vi "PPR_DRIVE_EXECUTE.vi"(6 "Pass_Through_Time":dbl=-1.0 format="%33.4f", 8 "error in (no error)":errorcluster) -> (0 "error out":errorcluster)   [LabVIEW 2019]
uses:
  <vilib>/Rock Robotics/WPI/ThirdParty/JAS_Junk/TrajLib/VI/BoolCmd_Recv_Internal.vi
  <vilib>/Rock Robotics/WPI/ThirdParty/JAS_Junk/TrajLib/VI/numCmd_ObtainQueue_TwoDbl.vi
  <vilib>/Rock Robotics/WPI/ThirdParty/JAS_Junk/TrajLib/VI/Util_GetTime_U32.vi
  <vilib>/Rock Robotics/WPI/ThirdParty/JAS_Junk/TrajLib/MathUtil_InputModulus.vi
  <vilib>/Rock Robotics/WPI/ThirdParty/JAS_Junk/TrajLib/VI/BoolCmd_ObtainQueue.vi
  <vilib>/Rock Robotics/WPI/ThirdParty/JAS_Junk/TrajLib/VI/Util_GetTime_U64.vi
  PPR_DRIVE_GLOBALS.vi
  <vilib>/Rock Robotics/WPI/ThirdParty/JAS_Junk/TrajLib/Trajectory_Library.lvlib
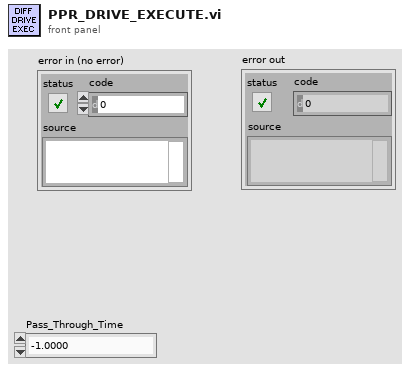
[diagram p1: front panel]
types:
  T1 = typedef "WPI_GyroDevRef.ctl" = cluster{"DevStatus":errorcluster, "Analog Channel":T2, "Gain (VoltsPerDegree/Second)":dbl, "Gyro Type":enum16{"Analog", "XRS450"}, "Handle":i32, "SPI Bus":T3, "Device Found":bool, "Sample Rate":dbl, "Calibrate On Open":bool, "Offset":dbl}
  T2 = typedef "FPGA_AIChannel.ctl" = enum8{"AI 0", "AI 1", "AI 2", "AI 3", "AI MXP 0", "AI MXP 1", "AI MXP 2", "AI MXP 3", "Invalid"}
  T3 = typedef "spi_bus.ctl" = enum16{"SPI On-Board, CS0", "SPI On-Board, CS1", "SPI On-Board, CS2", "SPI On-Board, CS3", "SPI MXP", "Invalid"}
  T4 = typedef "PPR_DRIVE_Wheel_TYPDEF.ctl" = cluster{"Drive Motor":T5, "Wheel Encoder":T10}
  T5 = typedef "WPI_MotorControlDeviceRef.ctl" = cluster{"DeviceStatus":errorcluster, "Type":T6, "PWM":cluster{"PWM Channel":T7, "DeadBand":T8}, "CAN":cluster{"Device Number":u8, "SetOutput VI Ref":variant, "GetOutput VI Ref":variant, "Enable VI Ref":variant, "Disable VI Ref":variant, "Data":variant}, "Invert":bool, "DIO PWM":cluster{"PWM \"Enable\" Channel":T7, "DIOChannel":T9, "PWM Rate":dbl}}
  T6 = typedef "WPI_MotorControlType.ctl" = enum16{"PWM", "CAN", "DIO PWM"}
  T7 = typedef "FPGA_DIOPWMChannel.ctl" = enum8{"PWM 0", "PWM 1", "PWM 2", "PWM 3", "PWM 4", "PWM 5", "PWM 6", "PWM 7", "PWM 8", "PWM 9", "PWM MXP 0", "PWM MXP 1", "PWM MXP 2", "PWM MXP 3", "PWM MXP 4", "PWM MXP 5", "PWM MXP 6", "PWM MXP 7", "PWM MXP 8", "PWM MXP 9", "Invalid"}
  T8 = typedef "WPI_PWMDeadband.ctl" = cluster{"Name":string, "maxPositivePwm":i32, "minPositivePwm":i32, "centerPwm":i32, "maxNegativePwm":i32, "minNegativePwm":i32, "angularRange":u16}
  T9 = typedef "FPGA_DIOChannel.ctl" = enum8{"DIO 0", "DIO 1", "DIO 2", "DIO 3", "DIO 4", "DIO 5", "DIO 6", "DIO 7", "DIO 8", "DIO 9", "DIO MXP 0", "DIO MXP 1", "DIO MXP 2", "DIO MXP 3", "DIO MXP 4", "DIO MXP 5", "DIO MXP 6", "DIO MXP 7", "DIO MXP 8", "DIO MXP 9", "DIO MXP 10", "DIO MXP 11", "DIO MXP 12", "DIO MXP 13", "DIO MXP 14", "DIO MXP 15", "SPI Port CS1", "SPI Port CS2", "SPI Port CS3", "SPI Port MISO", "SPI Port MOSI", "Invalid"}
  T10 = typedef "WPI_EncoderDevRef.ctl" = cluster{"DevStatus":errorcluster, "EncoderIndex":T11, "CounterIndex":T12, "DistancePerCount":dbl, "Decoding Type":T13}
  T11 = typedef "FPGA_EncoderIdx.ctl" = enum8{"Enc 0", "Enc 1", "Enc 2", "Enc 3", "Enc 4", "Enc 5", "Enc 6", "Enc 7", "Invalid"}
  T12 = typedef "FPGA_CounterCtrSystemIndex.ctl" = enum8{"Ctr 0", "Ctr 1", "Ctr 2", "Ctr 3", "Ctr 4", "Ctr 5", "Ctr 6", "Ctr 7", "Invalid"}
  T13 = typedef "WPI_EncoderType.ctl" = enum16{"1x", "2x", "4x"}
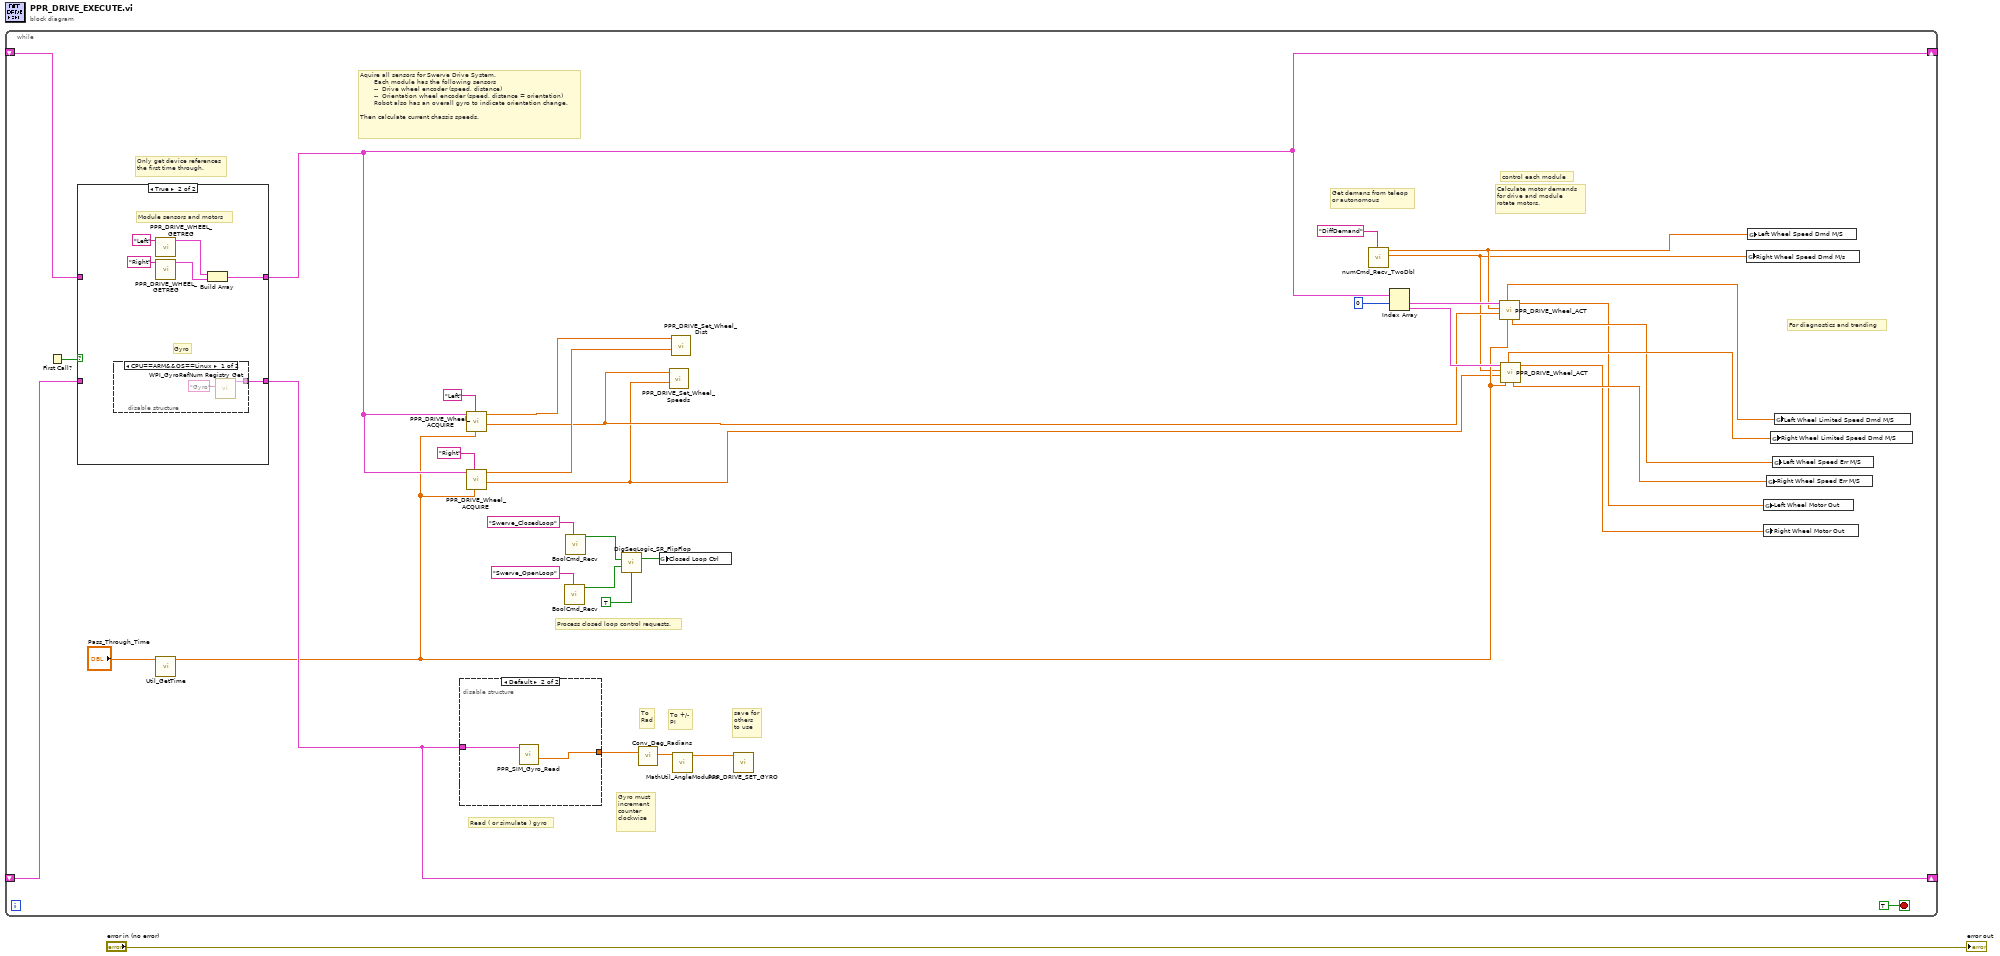
[diagram p0: block diagram]
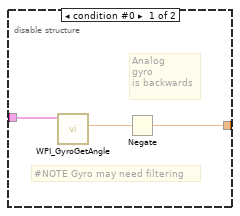
[diagram p4: hidden frame]
diagram:
  n1 = while {
    shift-right: [w25] -> _
    shift-left: _ -> [w26]
    shift-right: [w24] -> _
    shift-left: _ -> [w23]
    stop <- TRUE stop-if-true
    # "Process closed loop control requests."
    # "Only get device references\nthe first time through."
    # "save for\nothers\nto use"
    # "For diagnostics and trending"
    # "Gyro must\nincrement \ncounter\nclockwise"
    # "To +/-\nPI"
    # "To\nRad"
    # "Read ( or simulate ) gyro"
    # "Aquire all sensors for Swerve Drive System.\n       Each module has the following sensors\n       --  Drive wheel encoder (speed, distance)\n       --  Orientation wheel encoder (speed, distance = orientation)\n       Robot also has an overall gyro to indicate orientation change.\n\nThen calculate current chassis speeds."
    # "Calculate motor demands\nfor drive and module \nrotate motors."
    # "Get demans from teleop\nor autonomous"
    # "control each module"
    n2 = First Call?() -> (First Call?: T/F=w27:bool)
    n3 = case shown="True" w27 {
      tunnel: [w38 w42] -> w25
      tunnel: [w37 w41] -> w24
      tunnel: w26 -> [w38 _]
      tunnel: w23 -> [w37 _]
      frame False {
      }
      frame True {
        # "Module sensors and motors"
        # "Gyro"
        n4 = disable-structure shown="CPU==ARM&&OS==Linux" {
          disable-tunnel: [w45 _] -> w41
          frame condition #0 {
            n5 = call <vilib>:"WPI_GyroRefNum Registry Get.vi"("refnum name"="Gyro") -> ("GyroDevRef"=w45:T1)  [unwired: 9 in, 1 out]
          }
          frame condition #1 (active) {
          }
        }
        n6 = call "PPR_DRIVE_WHEEL_GETREG.vi"("Side"="Left") -> ("Diff Wheel TypDef"=w43:T4)  [unwired: 10 in]
        n7 = call "PPR_DRIVE_WHEEL_GETREG.vi"("Side"="Right") -> ("Diff Wheel TypDef"=w44:T4)  [unwired: 10 in]
        n8 = Build Array(w43, w44) -> (w42:T4[])
      }
    }
    n9 = call <vilib>:"Util_GetTime.vi"("Pass_Through_Time"="Pass_Through_Time") -> ("FPGA_Time_Seconds"=w22:dbl)  [unwired: 8 in, 2 out]
    n10 = disable-structure shown="Default" {
      disable-tunnel: w24 -> [w49 w51]
      disable-tunnel: [w47 w50] -> w30
      frame condition #0 {
        # "Analog\ngyro\nis backwards"
        # "#NOTE Gyro may need filtering"
        n11 = call <vilib>:"WPI_GyroGetAngle.vi"("GyroDevRef"=w49) -> ("Angle"=w48:dbl)  [unwired: 6 in, 4 out]
        n12 = Negate(x=w48) -> (-x=w47:dbl)
      }
      frame condition #1 (active) {
        n13 = call "PPR_SIM_Gyro_Read.vi"("GyroDevRef"=w51) -> ("Gyro_Cont_Deg"=w50:dbl)  [unwired: 10 in]
      }
    }
    n14 = call "PPR_DRIVE_Wheel_ACQUIRE.vi"("Pass_Through_Time"=w22, "Side"="Right", "Swerve Module TypDef"=w25) -> ("Speed M/S"=w10:dbl, "Distance M"=w12:dbl)  [unwired: 7 in]
    n15 = call "PPR_DRIVE_Wheel_ACQUIRE.vi"("Pass_Through_Time"=w22, "Side"="Left", "Swerve Module TypDef"=w25) -> ("Speed M/S"=w11:dbl, "Distance M"=w13:dbl)  [unwired: 7 in]
    n16 = call <vilib>:"BoolCmd_Recv.vi"("Command Name"="Swerve_OpenLoop") -> ("New Request"=w18:bool)  [unwired: 9 in, 1 out]
    n17 = call <vilib>:"BoolCmd_Recv.vi"("Command Name"="Swerve_ClosedLoop") -> ("New Request"=w19:bool)  [unwired: 9 in, 1 out]
    n18 = call <vilib>:"DigSeqLogic_SR_FlipFlop.vi"("Set"=w19, "Reset"=w18, "Initial Value"=TRUE) -> ("Output"=w16:bool)  [unwired: 11 in, 1 out]
    n19 = call <vilib>:"Conv_Deg_Radians.vi"("Degress"=w30) -> ("Radians"=w31:dbl)  [unwired: 10 in]
    n20 = global write "PPR_DRIVE_GLOBALS.vi" "Closed Loop Ctrl"(w16) -> ()
    n21 = call "PPR_DRIVE_Set_Wheel_Speeds.vi"("Right Wheel Speed M/S"=w10, "Left Wheel Speed M/S"=w11) -> ()  [unwired: 10 in]
    n22 = call "PPR_DRIVE_Set_Wheel_Dist.vi"("Right Wheel Dist M"=w12, "Left Wheel Dist M"=w13) -> ()  [unwired: 10 in]
    n23 = call <vilib>:"MathUtil_AngleModulus.vi"("InputAngle"=w31) -> ("ModulsAngle"=w29:dbl)  [unwired: 10 in]
    n24 = call "PPR_DRIVE_SET_GYRO.vi"("Gyro Heading Radians"=w29) -> ()  [unwired: 11 in]
    n25 = call <vilib>:"numCmd_Recv_TwoDbl.vi"("Command Name"="DiffDemand") -> ("Value 2"=w2:dbl, "Value 1"=w3:dbl)  [unwired: 7 in, 2 out]
    n26 = Index Array(array=w25, index #1=0 ("index")) -> (element #1=w34:T4, element #2=w35:T4)  [unwired: 1 in]
    n27 = call "PPR_DRIVE_Wheel_ACT.vi"("Pass_Through_Time"=w22, "Wheel Speed M/S"=w11, "Wheel Speed Dmd M/S"=w3, "Diff Wheel TypDef"=w34) -> ("Wheel Motor Dmd"=w5:dbl, "WheelSpeedErr"=w7:dbl, "Limited Speed Dmd M/S"=w9:dbl)  [unwired: 5 in]
    n28 = call "PPR_DRIVE_Wheel_ACT.vi"("Pass_Through_Time"=w22, "Wheel Speed M/S"=w10, "Wheel Speed Dmd M/S"=w2, "Diff Wheel TypDef"=w35) -> ("Wheel Motor Dmd"=w4:dbl, "WheelSpeedErr"=w6:dbl, "Limited Speed Dmd M/S"=w8:dbl)  [unwired: 5 in]
    n29 = global write "PPR_DRIVE_GLOBALS.vi" "Right Wheel Speed Dmd M/s"(w2) -> ()
    n30 = global write "PPR_DRIVE_GLOBALS.vi" "Left Wheel Speed Dmd M/S"(w3) -> ()
    n31 = global write "PPR_DRIVE_GLOBALS.vi" "Right Wheel Motor Out"(w4) -> ()
    n32 = global write "PPR_DRIVE_GLOBALS.vi" "Left Wheel Motor Out"(w5) -> ()
    n33 = global write "PPR_DRIVE_GLOBALS.vi" "Right Wheel Speed Err M/S"(w6) -> ()
    n34 = global write "PPR_DRIVE_GLOBALS.vi" "Right Wheel Limited Speed Dmd M/S"(w8) -> ()
    n35 = global write "PPR_DRIVE_GLOBALS.vi" "Left Wheel Speed Err M/S"(w7) -> ()
    n36 = global write "PPR_DRIVE_GLOBALS.vi" "Left Wheel Limited Speed Dmd M/S"(w9) -> ()
  }
  "error out" <- "error in (no error)"
